vi "CODMn通讯.vi"() -> ()   [LabVIEW 2016, in "斯坦道CODMn.lvlib"]
uses:
  <vilib>/NI/Modbus Library/API/Wrapper/Create TCP Slave.vi
  <vilib>/NI/Modbus Library/API/slave/Modbus Slave.lvclass
  <vilib>/Plasmionique/MB Master/MB_Master/MB_Master.lvclass
  <vilib>/Plasmionique/MB Master/MB Master.lvlib
  <vilib>/Utility/config.llb/NI_LVConfig.lvlib
  <vilib>/NI/Modbus Library/API/Wrapper/API Main.lvlib
panel:
  out "codm程序更新":bool=TRUE
  in  "读取数据":bool
  in  "释放串口":bool
  in  "打开串口":bool
  out "队列中元素数量":i32
  out "元素":cluster{"命令":string}[](array[cluster])
  out "待处理插入数量":i32
  out "读取公式":u16[](array[numeric])
  out "读取参数":u16[](array[numeric])
  out "数据存储":u16[](array[numeric])
  out "温度":bool[](array[boolean])
  out "M输出点":bool[](array[boolean])
  out "ORP、时间":u16[](array[numeric])
  out "测量状态":u16[](array[numeric])
  out "通讯状态":bool
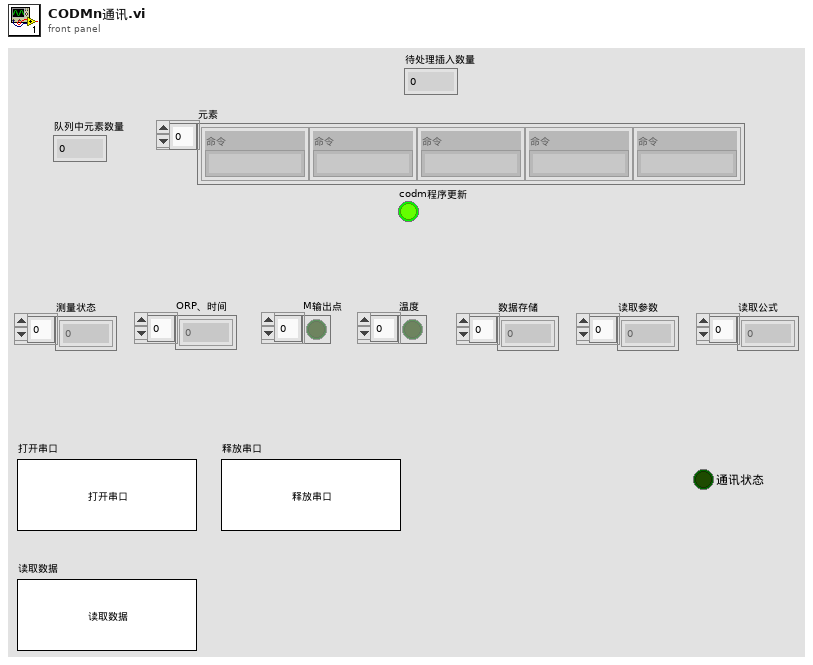
[diagram p1: front panel]
types:
  T1 = typedef "CODMn交互.ctl" = cluster{"COD浓度（mg/L)":dbl, "水样启动时间":timestamp, "加标回收启动时间":timestamp, "CODMn工作状态":enum16{"空闲", "水样测试", "标样核查", "零点核查", "跨度核查", "空白测试", "平行样测试", "加标回收", "空白校准", "标样校准", "初始化（清洗）"}, "多列列表框":i32, "平台试剂余量百分比":sgl, "关键参数":cluster{"测量量程":dbl, "测量精度":dbl, "测量间隔":dbl, "消解温度":dbl, "消解时长":dbl, "空白校准时间":timestamp, "曲线截距":dbl, "曲线斜率":dbl, "测量检出限":dbl, "测量信号值":dbl, "线性相关系数":dbl, "二次多项式系数":dbl, "标样校准时间":timestamp, "稀释倍数":dbl, "三项式系数":dbl, "空白标定系数":dbl, "量程系数":dbl, "F0/ORPA":dbl, "F1/ORPB":dbl, "F2/ORPK":dbl, "F3":dbl, "F4":dbl, "F5":dbl, "F6":dbl, "F7":dbl, "X0/滴定数":dbl, "量程":dbl}, "关键参数改变":bool, "校准信息":cluster{"低标液1浓度":dbl, "低标液1信号值":dbl, "低标液1启用":u16, "低标液2浓度":dbl, "低标液2信号值":dbl, "低标液2启用":u16, "低标液3浓度":dbl, "低标液3信号值":dbl, "低标液3启用":u16, "低标液4浓度":dbl, "低标液4信号值":dbl, "低标液4启用":u16, "低标液5浓度":dbl, "低标液5信号值":dbl, "低标液5启用":u16, "高标液1浓度":dbl, "高标液1信号值":dbl, "高标液1启用":u16, "高标液2浓度":dbl, "高标液2信号值":dbl, "高标液2启用":u16, "高标液3浓度":dbl, "高标液3信号值":dbl, "高标液3启用":u16, "高标液4浓度":dbl, "高标液4信号值":dbl, "高标液4启用":u16, "高标液5浓度":dbl, "高标液5信号值":dbl, "高标液5启用":u16}, "校准信息改变":bool}
  T2 = cluster{"测量模式":enum16{"水样测量", "标样核查", "零点核查", "跨度核查", "空白测试", "加标回收", "平行样", "校零", "校标"}}
  T3 = cluster{"命令":string, "测量模式":enum16{"水样测量", "标样核查", "零点核查", "跨度核查", "空白测试", "加标回收", "平行样", "校零", "校标"}, "CODMn量程切换":enum32{"H", "L", "AUTO"}}
  T4 = typedef "NI_LVConfig.lvlib/Config Data RefNum.ctl" = refnum<k1>
  T5 = enum16{"空闲", "水样测试", "标样核查", "零点核查", "跨度核查", "空白测试", "平行样测试", "质控样", "空白校准", "标样校准", "加标回收"}
  T6 = cluster{"测量量程":dbl, "测量精度":dbl, "测量间隔":dbl, "消解温度":dbl, "消解时长":dbl, "空白校准时间":timestamp, "曲线截距":dbl, "曲线斜率":dbl, "测量检出限":dbl, "测量信号值":dbl, "线性相关系数":dbl, "二次多项式系数":dbl, "标样校准时间":timestamp, "稀释倍数":dbl, "三项式系数":dbl, "空白标定系数":dbl, "量程系数":dbl, "F0/ORPA":dbl, "F1/ORPB":dbl, "F2/ORPK":dbl, "F3":dbl, "F4":dbl, "F5":dbl, "F6":dbl, "F7":dbl, "X0/滴定数":dbl, "量程":dbl}
  T7 = cluster{"低标液1浓度":dbl, "低标液1信号值":dbl, "低标液1启用":u16, "低标液2浓度":dbl, "低标液2信号值":dbl, "低标液2启用":u16, "低标液3浓度":dbl, "低标液3信号值":dbl, "低标液3启用":u16, "低标液4浓度":dbl, "低标液4信号值":dbl, "低标液4启用":u16, "低标液5浓度":dbl, "低标液5信号值":dbl, "低标液5启用":u16, "高标液1浓度":dbl, "高标液1信号值":dbl, "高标液1启用":u16, "高标液2浓度":dbl, "高标液2信号值":dbl, "高标液2启用":u16, "高标液3浓度":dbl, "高标液3信号值":dbl, "高标液3启用":u16, "高标液4浓度":dbl, "高标液4信号值":dbl, "高标液4启用":u16, "高标液5浓度":dbl, "高标液5信号值":dbl, "高标液5启用":u16}
  T8 = enum16{"水样测量", "标样核查", "零点核查", "跨度核查", "空白测试", "加标回收", "平行样", "校零", "校标"}
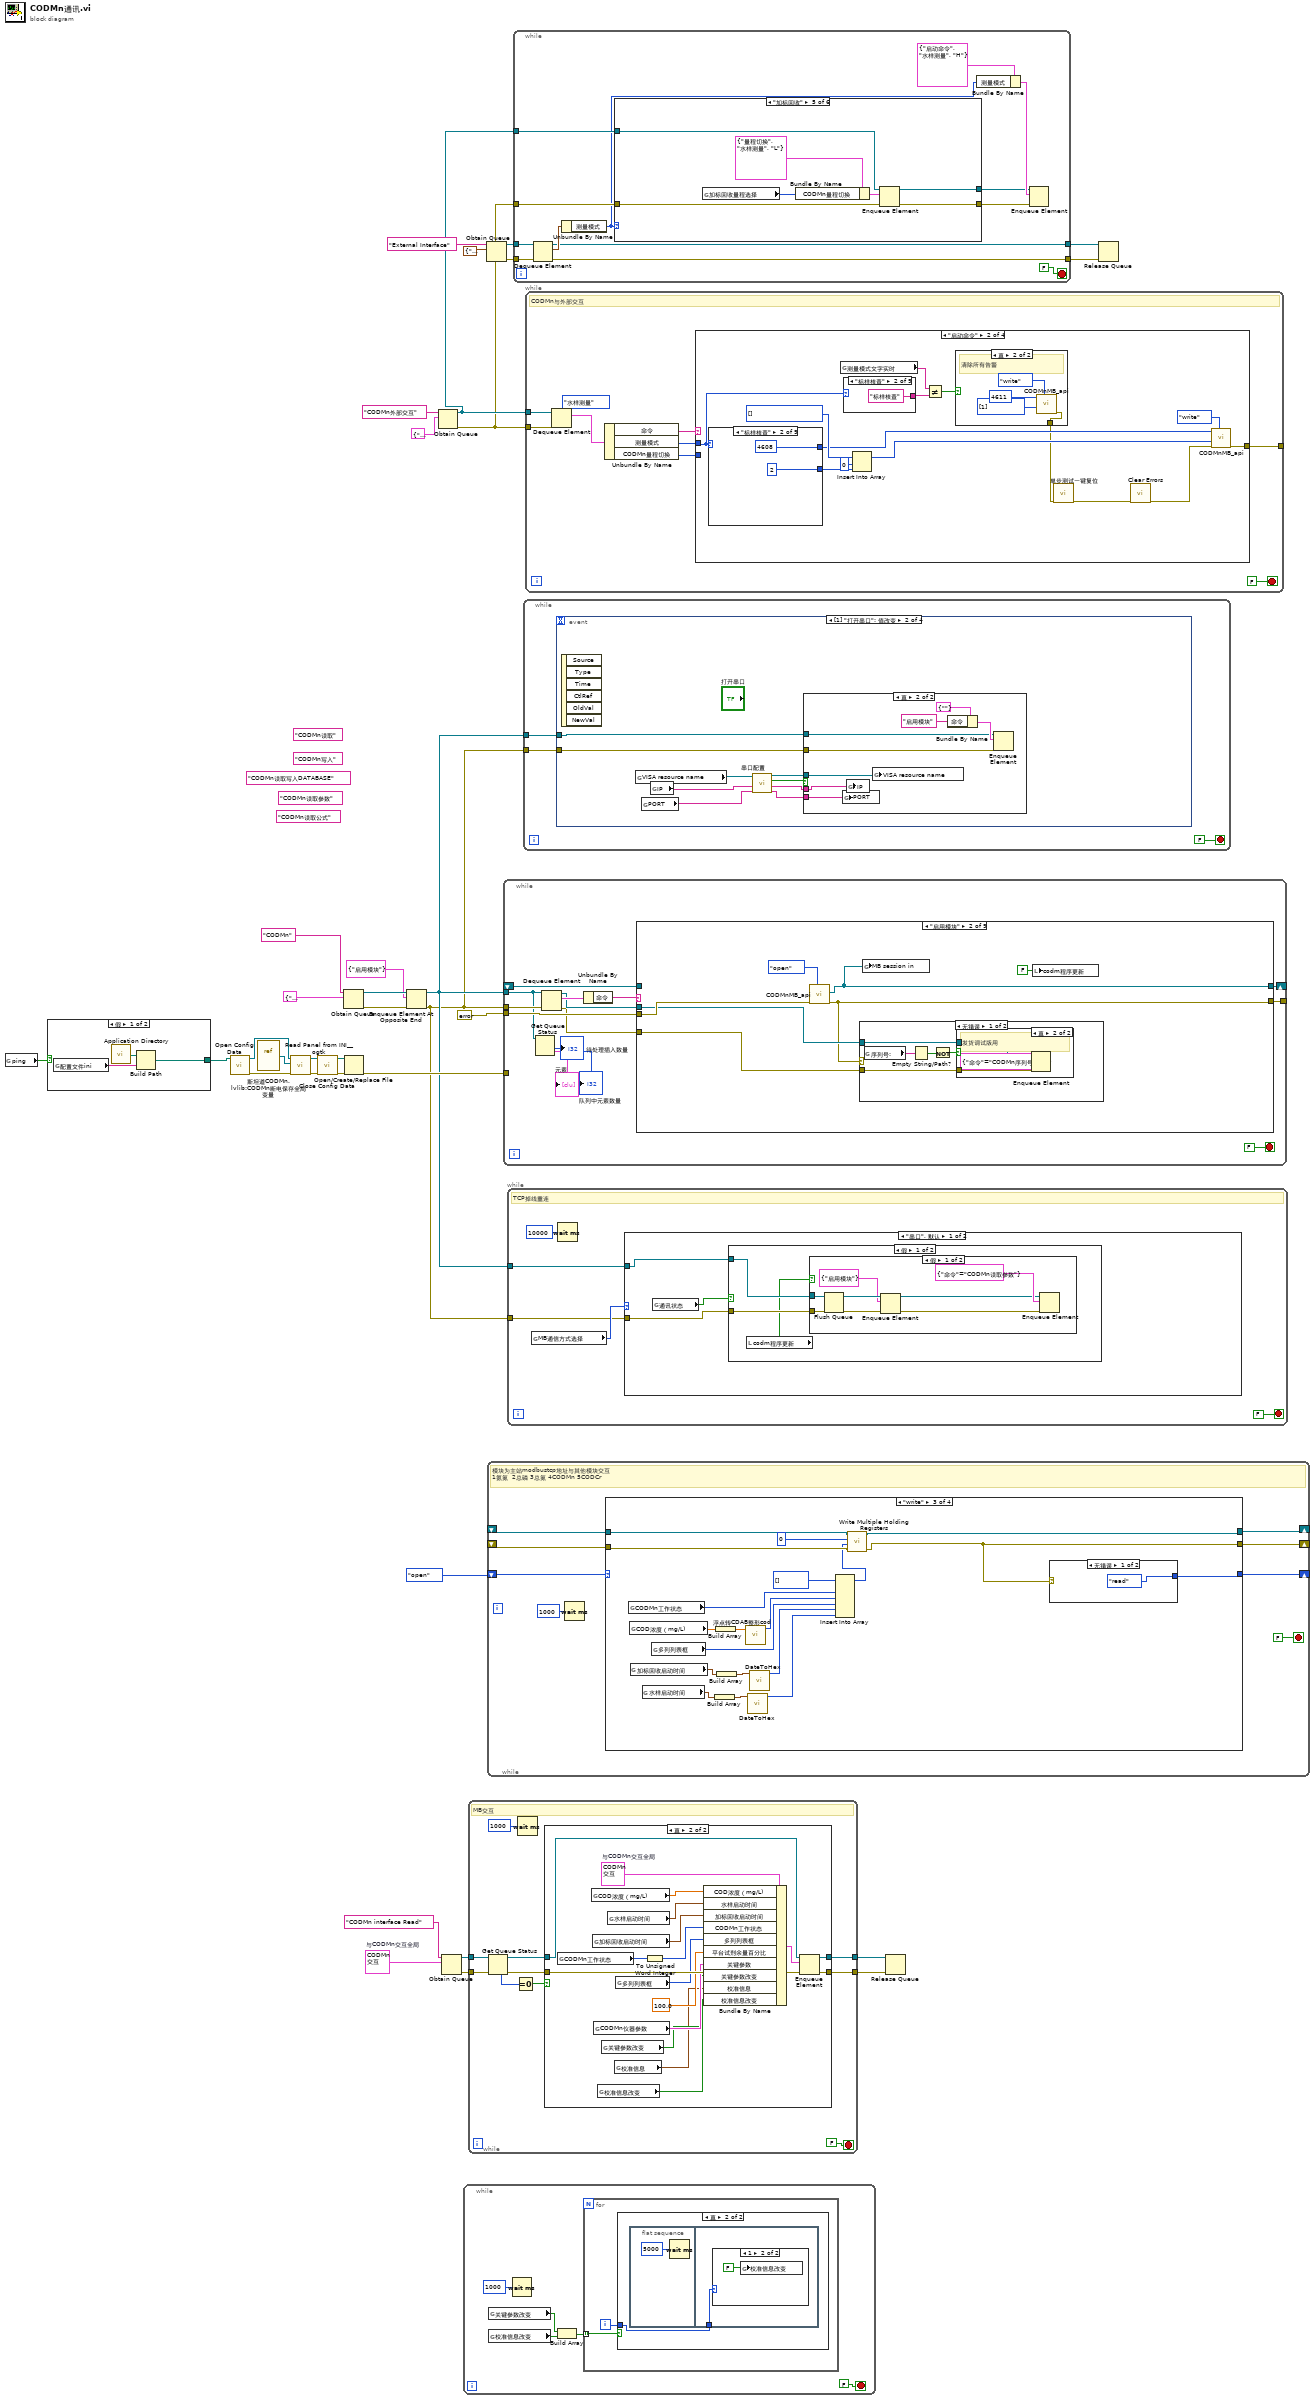
[diagram p0: block diagram]
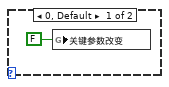
[diagram p3: hidden frame]
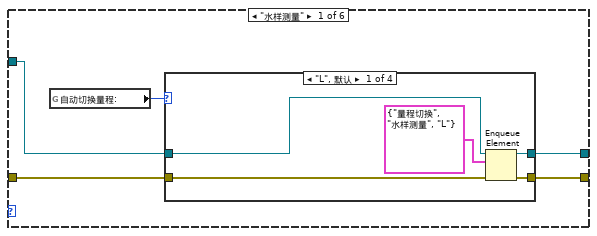
[diagram p5: hidden frame]
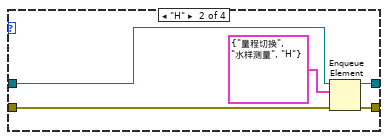
[diagram p6: hidden frame]
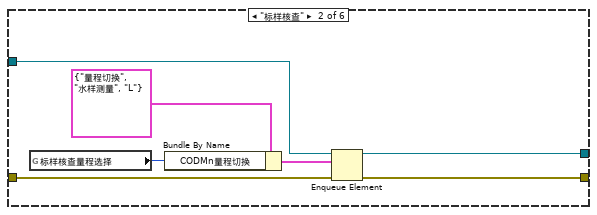
[diagram p9: hidden frame]
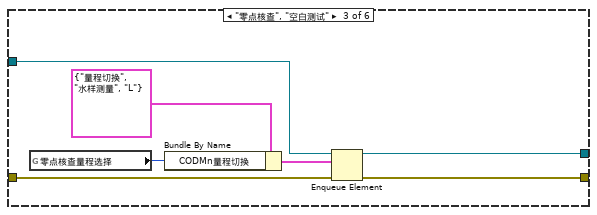
[diagram p10: hidden frame]
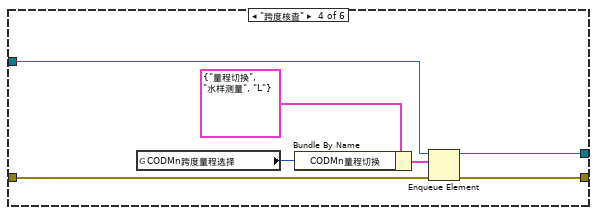
[diagram p11: hidden frame]
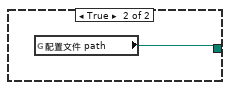
[diagram p13: hidden frame]
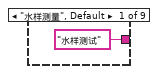
[diagram p16: hidden frame]
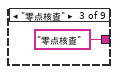
[diagram p17: hidden frame]
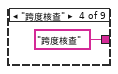
[diagram p18: hidden frame]
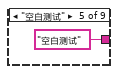
[diagram p19: hidden frame]
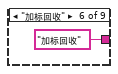
[diagram p20: hidden frame]
diagram:
  w2 = T1 {"COD浓度（mg/L)"=0.0, "水样启动时间"=timestamp(0 s since 1904-01-01), "加标回收启动时间"=timestamp(0 s since 1904-01-01), "CODMn工作状态"=enum."空闲", "多列列表框"=0, "平台试剂余量百分比"=0.0, "关键参数"={"测量量程"=0.0, "测量精度"=0.0, "测量间隔"=0.0, "消解温度"=0.0, "消解时长"=0.0, "空白校准时间"=timestamp(0 s since 1904-01-01), "曲线截距"=0.0, "曲线斜率"=0.0, "测量检出限"=0.0, "测量信号值"=0.0, "线性相关系数"=0.0, "二次多项式系数"=0.0, "标样校准时间"=timestamp(0 s since 1904-01-01), "稀释倍数"=0.0, "三项式系数"=0.0, "空白标定系数"=0.0, "量程系数"=0.0, "F0/ORPA"=0.0, "F1/ORPB"=0.0, "F2/ORPK"=0.0, "F3"=0.0, "F4"=0.0, "F5"=0.0, "F6"=0.0, "F7"=0.0, "X0/滴定数"=0.0, "量程"=0.0}, "关键参数改变"=FALSE, "校准信息"={"低标液1浓度"=0.0, "低标液1信号值"=0.0, "低标液1启用"=0, "低标液2浓度"=0.0, "低标液2信号值"=0.0, "低标液2启用"=0, "低标液3浓度"=0.0, "低标液3信号值"=0.0, "低标液3启用"=0, "低标液4浓度"=0.0, "低标液4信号值"=0.0, "低标液4启用"=0, "低标液5浓度"=0.0, "低标液5信号值"=0.0, "低标液5启用"=0, "高标液1浓度"=0.0, "高标液1信号值"=0.0, "高标液1启用"=0, "高标液2浓度"=0.0, "高标液2信号值"=0.0, "高标液2启用"=0, "高标液3浓度"=0.0, "高标液3信号值"=0.0, "高标液3启用"=0, "高标液4浓度"=0.0, "高标液4信号值"=0.0, "高标液4启用"=0, "高标液5浓度"=0.0, "高标液5信号值"=0.0, "高标液5启用"=0}, "校准信息改变"=FALSE}  # 与CODMn交互全局
  (unwired) "CODMn读取公式" ("名称（未命名）")
  (unwired) "CODMn读取写入DATABASE" ("名称（未命名）")
  (unwired) "CODMn读取参数" ("名称（未命名）")
  (unwired) "CODMn读取" ("名称（未命名）")
  (unwired) "CODMn写入" ("名称（未命名）")
  n1 = global read "CODMN外部API.vi" "ping"() -> (w17:bool)
  n2 = case shown="假" w17 {
    tunnel: [w36 w39] -> w16
    frame False {
      n3 = global read "COD内部交互全局.vi" "配置文件ini"() -> (w38:string)
      n4 = call <vilib>:"Application Directory.vi"() -> ("Application Directory"=w37:path)
      n5 = Build Path(base path=w37, name or relative path=w38) -> (appended path=w36:path)
    }
    frame True {
      n6 = global read "CODMN外部API.vi" "配置文件 path"() -> (w39:path)
    }
  }
  n7 = call <vilib>:"Open Config Data.vi"("configuration file path"=w16) -> ("error out"=w27:errorcluster, "refnum"=w30:T4)  [unwired: 8 in, 1 out]
  n8 = vi-ref "斯坦道CODMn.lvlib:CODMn断电保存全局变量.vi"() -> (w29:refnum<vi>)
  n9 = call <userlib>:"Read Panel from INI__ogtk.vi"("error in (no error)"=w27, "VI ref"=w29, "refnum"=w30) -> ("error out"=w26:errorcluster, "refnum out"=w28:T4)  [unwired: 7 in]
  n10 = call <vilib>:"Close Config Data.vi"("error in (no error)"=w26, "refnum"=w28) -> ("error out"=w25:errorcluster, "file path"=w24:path)  [unwired: 8 in]
  n11 = Obtain Queue(name (unnamed)="CODMn", element data type=cluster{"命令":string} {"命令"="启用模块"} ("元素")) -> (queue out=w33:refnum<queue>, error out=w32:errorcluster)  [unwired: 3 in, 1 out]
  n12 = Open/Create/Replace File(file path (use dialog)=w24, error in=w25) -> (error out=w23:errorcluster)  [unwired: 4 in, 2 out]
  n13 = Enqueue Element At Opposite End(queue=w33, element=cluster{"命令":string} {"命令"="启用模块"} ("元素"), error in (no error)=w32) -> (queue out=w21:refnum<queue>, error out=w20:errorcluster)  [unwired: 1 in, 1 out]
  n14 = Obtain Queue(name (unnamed)="CODMn外部交互" ("名称（未命名）"), element data type=T3 {"命令"="启动命令", "测量模式"=enum."水样测量", "CODMn量程切换"=enum."AUTO"} ("元素")) -> (queue out=w11:refnum<queue>, error out=w10:errorcluster)  [unwired: 3 in, 1 out]
  n15 = Obtain Queue(name (unnamed)="CODMn interface Read" ("写入方名称"), element data type=w2) -> (queue out=w6:refnum<queue>, error out=w5:errorcluster)  [unwired: 3 in, 1 out]
  n16 = while {
    stop <- FALSE stop-if-true
    n17 = global read "CODMn断电保存全局变量.vi" "关键参数改变"() -> (w43:bool)
    n18 = global read "CODMn断电保存全局变量.vi" "校准信息改变"() -> (w42:bool)
    n19 = Wait (ms)(milliseconds to wait=u32 1000 ("等待时间（毫秒）")) -> ()  [unwired: 1 out]
    n20 = Build Array(w43, w42) -> (w41:bool[])
    n21 = for {
      tunnel: w41 -> [w46] mode=indexing
      i -> [w45]
      n22 = case shown="真" w46 {
        tunnel: w45 -> [_ w47]
        frame False {
        }
        frame True {
          n23 = flat-sequence {
            tunnel: w47 -> [w49]
            frame #0 {
              n24 = Wait (ms)(milliseconds to wait=u32 5000 ("等待时间（毫秒）")) -> ()  [unwired: 1 out]
            }
            frame #1 {
              n25 = case shown="1" w49 {
                frame 0, Default {
                  n26 = global write "CODMn断电保存全局变量.vi" "关键参数改变"(FALSE ("关键参数改变")) -> ()
                }
                frame 1 {
                  n27 = global write "CODMn断电保存全局变量.vi" "校准信息改变"(FALSE ("关键参数改变")) -> ()
                }
              }
            }
          }
        }
      }
    }
  }
  n28 = while {
    tunnel: w6 -> [w60]
    tunnel: w5 -> [w53]
    tunnel: [w59] -> w4
    tunnel: [w58] -> w3
    stop <- FALSE stop-if-true
    # "MB交互"
    n29 = Get Queue Status(queue=w60, error in (no error)=w53) -> (queue out=w56:refnum<queue>, error out=w52:errorcluster, # elements in queue=w55:i32)  [unwired: 1 in, 5 out]
    n30 = Equal To 0?(x=w55) -> (x = 0?=w54:bool)
    n31 = Wait (ms)(milliseconds to wait=u32 1000 ("等待时间（毫秒）")) -> ()  [unwired: 1 out]
    n32 = case shown="真" w54 {
      tunnel: w56 -> [w63 w80]
      tunnel: w52 -> [w62 w79]
      tunnel: [w63 w78] -> w59
      tunnel: [w62 w77] -> w58
      frame False {
      }
      frame True {
        w76 = T1 {"COD浓度（mg/L)"=0.0, "水样启动时间"=timestamp(0 s since 1904-01-01), "加标回收启动时间"=timestamp(0 s since 1904-01-01), "CODMn工作状态"=enum."空闲", "多列列表框"=0, "平台试剂余量百分比"=0.0, "关键参数"={"测量量程"=0.0, "测量精度"=0.0, "测量间隔"=0.0, "消解温度"=0.0, "消解时长"=0.0, "空白校准时间"=timestamp(0 s since 1904-01-01), "曲线截距"=0.0, "曲线斜率"=0.0, "测量检出限"=0.0, "测量信号值"=0.0, "线性相关系数"=0.0, "二次多项式系数"=0.0, "标样校准时间"=timestamp(0 s since 1904-01-01), "稀释倍数"=0.0, "三项式系数"=0.0, "空白标定系数"=0.0, "量程系数"=0.0, "F0/ORPA"=0.0, "F1/ORPB"=0.0, "F2/ORPK"=0.0, "F3"=0.0, "F4"=0.0, "F5"=0.0, "F6"=0.0, "F7"=0.0, "X0/滴定数"=0.0, "量程"=0.0}, "关键参数改变"=FALSE, "校准信息"={"低标液1浓度"=0.0, "低标液1信号值"=0.0, "低标液1启用"=0, "低标液2浓度"=0.0, "低标液2信号值"=0.0, "低标液2启用"=0, "低标液3浓度"=0.0, "低标液3信号值"=0.0, "低标液3启用"=0, "低标液4浓度"=0.0, "低标液4信号值"=0.0, "低标液4启用"=0, "低标液5浓度"=0.0, "低标液5信号值"=0.0, "低标液5启用"=0, "高标液1浓度"=0.0, "高标液1信号值"=0.0, "高标液1启用"=0, "高标液2浓度"=0.0, "高标液2信号值"=0.0, "高标液2启用"=0, "高标液3浓度"=0.0, "高标液3信号值"=0.0, "高标液3启用"=0, "高标液4浓度"=0.0, "高标液4信号值"=0.0, "高标液4启用"=0, "高标液5浓度"=0.0, "高标液5信号值"=0.0, "高标液5启用"=0}, "校准信息改变"=FALSE}  # 与CODMn交互全局
        n33 = global read "COD测量模式全局.vi" "CODMn工作状态"() -> (w73:T5)
        n34 = global read "COD浓度全局变量.vi" "COD浓度（mg/L)"() -> (w68:dbl)
        n35 = global read "COD测量模式全局.vi" "加标回收启动时间"() -> (w72:timestamp)
        n36 = global read "CODMn断电保存全局变量.vi" "CODMn仪器参数"() -> (w75:T6)
        n37 = global read "CODMn断电保存全局变量.vi" "校准信息改变"() -> (w65:bool)
        n38 = global read "CODMn断电保存全局变量.vi" "关键参数改变"() -> (w66:bool)
        n39 = global read "COD测量模式全局.vi" "水样启动时间"() -> (w71:timestamp)
        n40 = global read "CODMn断电保存全局变量.vi" "校准信息"() -> (w64:T7)
        n41 = global read "运行时序全局变量.vi" "多列列表框"() -> (w69:i32)
        n42 = To Unsigned Word Integer(number=w73) -> (unsigned 16bit integer=w74:u16)
        n43 = Bundle By Name(cluster=w76, "COD浓度（mg/L)"=w68, "水样启动时间"=w71, "加标回收启动时间"=w72, "CODMn工作状态"=w74, "多列列表框"=w69, "平台试剂余量百分比"=sgl 100.0, "关键参数"=w75, "关键参数改变"=w66, "校准信息"=w64, "校准信息改变"=w65) -> (w67:T1)
        n44 = Enqueue Element(queue=w80, element=w67, error in (no error)=w79) -> (queue out=w78:refnum<queue>, error out=w77:errorcluster)  [unwired: 1 in, 1 out]
      }
    }
  }
  n45 = Obtain Queue(name (unnamed)="External Interface" ("名称（未命名）"), element data type=T2 {"测量模式"=enum."水样测量"} ("启动测量模式")) -> (queue out=w13:refnum<queue>, error out=w12:errorcluster)  [unwired: 3 in, 1 out]
  n46 = while {
    shift-right: [w86] -> _
    shift-left: _ -> [w88]
    shift-right: [w85] -> _
    shift-left: _ -> [w87]
    shift-right: [w82] -> _
    shift-left: enum16{"open", "read", "write", "close"}."open" -> [w83]
    stop <- FALSE stop-if-true
    # "模块为主站modbustcp地址与其他模块交互\n1氨氮  2总磷 3总氮 4CODMn 5CODCr"
    n47 = Wait (ms)(milliseconds to wait=u32 1000 ("等待时间（毫秒）")) -> ()  [unwired: 1 out]
    n48 = case shown="\"write\"" w83 {
      selector: w83 -> [w97 _ _ _]
      tunnel: w88 -> [w91 w105 w128 w134]
      tunnel: w87 -> [w90 w104 w125 w133]
      tunnel: [w94 w101 w127 w134] -> w86
      tunnel: [w93 w100 w126 w136] -> w85
      tunnel: [w96 w108 w129 enum16{"open", "read", "write", "close"}."open"] -> w82
      frame "open", Default {
        n49 = call-dynamic "Shutdown.vi"("error in"=w90, "Modbus slave in"=w91) -> ("error out"=w89:errorcluster)  [unwired: 9 in]
        n50 = call <vilib>:"Clear Errors.vi"("error in (no error)"=w89) -> ("error out"=w92:errorcluster)  [unwired: 5 in, 1 out]
        n51 = call-poly <vilib>:"Create Modbus Instance.vi"("error in"=w92, "port (502)"=u16 4) -> ("error out"=w93:errorcluster, "TCP slave instance"=w94:refnum<class "Modbus Slave.lvclass">)  [unwired: 8 in]
        n52 = case shown="错误" w93 {
          tunnel: w97 -> [_ w99]
          tunnel: [enum16{"open", "read", "write", "close"}."write" w99] -> w96
          frame No Error {
          }
          frame Error {
          }
        }
      }
      frame "read" {
        n53 = call-dynamic <vilib>:"Read Holding Registers.vi"("error in"=w104, "number of inputs"=u16 1, "starting address"=u16 257, "Modbus slave in"=w105) -> ("error out"=w100:errorcluster, "register values"=w103:u16[], "Modbus slave out"=w101:refnum<class "Modbus Slave.lvclass">)  [unwired: 5 in]
        n54 = Index Array(array=w103) -> (element=w102:u16)  [unwired: 1 in]
        n55 = global write "CODMN外部API.vi" "CODMn状态"(w102) -> ()
        n56 = case shown="无错误" w100 {
          tunnel: [enum16{"open", "read", "write", "close"}."write" enum16{"open", "read", "write", "close"}."close"] -> w108
          frame No Error {
          }
          frame Error {
          }
        }
      }
      frame "write" {
        n57 = global read "COD测量模式全局.vi" "CODMn工作状态"() -> (w115:T5)
        n58 = global read "COD浓度全局变量.vi" "COD浓度（mg/L)"() -> (w117:dbl)
        n59 = global read "COD测量模式全局.vi" "加标回收启动时间"() -> (w120:timestamp)
        n60 = global read "COD测量模式全局.vi" "水样启动时间"() -> (w122:timestamp)
        n61 = global read "运行时序全局变量.vi" "多列列表框"() -> (w119:i32)
        n62 = Build Array(w122) -> (w121:timestamp[])
        n63 = Build Array(w117) -> (w116:dbl[])
        n64 = Build Array(w120) -> (w113:timestamp[])
        n65 = call "浮点转CDAB整形cod.vi"("浮点数"=w116) -> ("CDAB整形输出"=w118:u16[])  [unwired: 10 in]
        n66 = call "DateToHex.vi"("DATE"=w121) -> ("数组"=w124:u16[])  [unwired: 10 in]
        n67 = call "DateToHex.vi"("DATE"=w113) -> ("数组"=w123:u16[])  [unwired: 10 in]
        n68 = Insert Into Array(array=u16[] [] ("values"), new element #1=w115, new element #2=w118, new element #3=w119, new element #4=w123, new element #5=w124) -> (w112:u16[])  [unwired: 1 in]
        n69 = call-dynamic "Write Multiple Holding Registers.vi"("error in"=w125, "registers to write"=w112, "starting address"=u16 0, "Modbus slave in"=w128) -> ("error out"=w126:errorcluster, "Modbus slave out"=w127:refnum<class "Modbus Slave.lvclass">)  [unwired: 6 in]
        n70 = case shown="无错误" w126 {
          tunnel: [enum16{"open", "read", "write", "close"}."read" enum16{"open", "read", "write", "close"}."close"] -> w129
          frame No Error {
          }
          frame Error {
          }
        }
      }
      frame "close" {
        n71 = call-dynamic "Shutdown.vi"("error in"=w133, "Modbus slave in"=w134) -> ("error out"=w132:errorcluster)  [unwired: 9 in]
        n72 = call <vilib>:"Clear Errors.vi"("error in (no error)"=w132) -> ("error out"=w136:errorcluster)  [unwired: 5 in, 1 out]
      }
    }
  }
  n73 = while {
    tunnel: w21 -> [w142]
    tunnel: w20 -> [w149]
    tunnel: [w143] -> _
    shift-right: [w146] -> _
    shift-left: _ -> [w145]
    tunnel: errorcluster {"status"=FALSE, "code"=0, "source"=""} ("error out") -> [w144]
    tunnel: w23 -> [_]
    stop <- FALSE stop-if-true
    n74 = Get Queue Status(queue=w142) -> (# pending insert=→"待处理插入数量":i32, # elements in queue=→"队列中元素数量":i32, elements=→"元素":cluster{"命令":string}[])  [unwired: 2 in, 5 out]
    n75 = Dequeue Element(queue=w142, error in (no error)=w149) -> (queue out=w138:refnum<queue>, element=w148:cluster{"命令":string}, error out=w137:errorcluster)  [unwired: 1 in, 1 out]
    n76 = Unbundle By Name(w148) -> ("命令"=w147:string)
    n77 = case shown="\"启用模块\"" w147 {
      tunnel: [w152 w157 w169 w177 w209 w218 w235 w242 w249] -> w146
      tunnel: [w151 w154 w170 w174 w207 w217 w234 w241 w248] -> w143
      tunnel: w145 -> [w152 _ _ w201 w213 w227 w238 w246 w252]
      tunnel: w144 -> [w151 w158 w171 w200 w210 w226 w237 w245 w250]
      tunnel: w138 -> [_ w156 _ _ _ _ _ _ _]
      tunnel: w137 -> [_ w155 _ _ _ _ _ _ _]
      frame Default {
      }
      frame "启用模块" {
        n78 = call "CODMnMB_api.vi"("STEP"=enum16{"open", "read", "write", "close"}."open", "Error in"=w158) -> ("error out"=w154:errorcluster, "MB session out"=w157:refnum<class "MB_Master.lvclass">)  [unwired: 7 in, 1 out]
        n79 = case shown="无错误" w154 {
          tunnel: w156 -> [w164 _]
          tunnel: w155 -> [w163 _]
          frame No Error {
            n80 = global read "COD内部交互全局.vi" "序列号:"() -> (w162:string)
            n81 = Empty String/Path?(string/path=w162) -> (empty?=w161:bool)
            n82 = Not(x=w161) -> (.not. x?=w160:bool)
            n83 = case shown="真" w160 {
              tunnel: w164 -> [_ w167]
              tunnel: w163 -> [_ w166]
              frame False {
              }
              frame True {
                # "发货调试版用"
                n84 = Enqueue Element(queue=w167, element=cluster{"命令":string} {"命令"="CODMn序列号写入"} ("元素"), error in (no error)=w166) -> ()  [unwired: 1 in, 3 out]
              }
            }
          }
          frame Error {
          }
        }
        n85 = global write "COD浓度全局变量.vi" "MB session in"(w157) -> ()
        n86 = local write "codm程序更新"(FALSE ("codm程序更新")) -> ()
      }
      frame "停用模块" {
        n87 = call "CODMnMB_api.vi"("STEP"=enum16{"open", "read", "write", "close"}."close", "Error in"=w171) -> ("error out"=w170:errorcluster, "MB session out"=w169:refnum<class "MB_Master.lvclass">)  [unwired: 7 in, 1 out]
        "codm程序更新" <- TRUE
      }
      frame "CODMn读取" {
        n88 = call <vilib>:"Read Holding Registers.vi"("error in (no error)"=w200, "quantity"=u16 50 ("number of holding registers"), "starting address"=u16 4224, "MB session in"=w201) -> ("error out"=w191:errorcluster, "Registers"=w197:u16[], "MB session out"=w192:refnum<class "MB_Master.lvclass">)  [unwired: 5 in]
        n89 = case shown="无错误" w191 {
          tunnel: w197 -> [w206 _]
          frame No Error {
            n90 = global write "COD内部交互全局.vi" "测量状态"(w206) -> ()
            "测量状态" <- w206
          }
          frame Error {
          }
        }
        n91 = call <vilib>:"Read Holding Registers.vi"("error in (no error)"=w191, "quantity"=u16 10, "starting address"=u16 4101, "MB session in"=w192) -> ("error out"=w187:errorcluster, "Registers"=w190:u16[], "MB session out"=w189:refnum<class "MB_Master.lvclass">)  [unwired: 5 in]
        n92 = case shown="无错误" w187 {
          tunnel: w190 -> [w205 _]
          frame No Error {
            n93 = global write "COD内部交互全局.vi" "ORP、时间"(w205) -> ()
            "ORP、时间" <- w205
          }
          frame Error {
          }
        }
        n94 = call <vilib>:"Read Coils.vi"("error in (no error)"=w187, "quantity"=u16 11, "starting address"=u16 137, "MB session in"=w189) -> ("error out"=w185:errorcluster, "Coils"=w186:bool[], "MB session out"=w188:refnum<class "MB_Master.lvclass">)  [unwired: 5 in]
        n95 = case shown="无错误" w185 {
          tunnel: w186 -> [w204 _]
          frame No Error {
            n96 = global write "COD内部交互全局.vi" "M输出点"(w204) -> ()
            "M输出点" <- w204
          }
          frame Error {
          }
        }
        n97 = call <vilib>:"Read Coils.vi"("error in (no error)"=w185, "quantity"=u16 1, "starting address"=u16 400, "MB session in"=w188) -> ("error out"=w178:errorcluster, "Coils"=w182:bool[], "MB session out"=w179:refnum<class "MB_Master.lvclass">)  [unwired: 5 in]
        n98 = case shown="无错误" w178 {
          tunnel: w182 -> [w203 _]
          frame No Error {
            n99 = global write "COD内部交互全局.vi" "温度"(w203) -> ()
            "温度" <- w203
          }
          frame Error {
          }
        }
        n100 = call <vilib>:"Read Coils.vi"("error in (no error)"=w178, "quantity"=u16 20, "starting address"=u16 500, "MB session in"=w179) -> ("error out"=w174:errorcluster, "Coils"=w173:bool[], "MB session out"=w177:refnum<class "MB_Master.lvclass">)  [unwired: 5 in]
        n101 = case shown="无错误" w174 {
          tunnel: w173 -> [w202 _]
          frame No Error {
            n102 = global write "COD内部交互全局.vi" "报警点位"(w202) -> ()
          }
          frame Error {
          }
        }
        n103 = Unbundle By Name(w174) -> ("status"=w181:bool)
        n104 = Not(x=w181) -> (.not. x?=w180:bool)
        "通讯状态" <- w180
        n105 = global write "COD内部交互全局.vi" "通讯状态"(w180) -> ()
      }
      frame "CODMn读取写入DATABASE" {
        n106 = call <vilib>:"Read Holding Registers.vi"("error in (no error)"=w210, "quantity"=u16 10 ("number of holding registers"), "starting address"=u16 4101, "MB session in"=w213) -> ("error out"=w207:errorcluster, "Registers"=w208:u16[], "MB session out"=w209:refnum<class "MB_Master.lvclass">)  [unwired: 5 in]
        n107 = case shown="无错误" w207 {
          tunnel: w208 -> [w215 _]
          frame No Error {
            n108 = global write "COD内部交互全局.vi" "数据存储"(w215) -> ()
            n109 = global write "COD内部交互全局.vi" "读取写入data"(TRUE ("读取参数显示")) -> ()
            "数据存储" <- w215
          }
          frame Error {
          }
        }
      }
      frame "CODMn读取参数" {
        n110 = call <vilib>:"Read Holding Registers.vi"("error in (no error)"=w226, "quantity"=u16 35 ("number of holding registers"), "starting address"=u16 4272, "MB session in"=w227) -> ("error out"=w221:errorcluster, "Registers"=w223:u16[], "MB session out"=w222:refnum<class "MB_Master.lvclass">)  [unwired: 5 in]
        n111 = case shown="无错误" w221 {
          tunnel: w223 -> [w231 _]
          frame No Error {
            n112 = global write "COD内部交互全局.vi" "读取参数"(w231) -> ()
            n113 = global write "COD内部交互全局.vi" "读取参数显示"(TRUE ("读取参数显示")) -> ()
            "读取参数" <- w231
          }
          frame Error {
          }
        }
        n114 = call <vilib>:"Read Holding Registers.vi"("error in (no error)"=w221, "quantity"=u16 4, "starting address"=u16 5596, "MB session in"=w222) -> ("error out"=w217:errorcluster, "Registers"=w216:u16[], "MB session out"=w218:refnum<class "MB_Master.lvclass">)  [unwired: 5 in]
        n115 = case shown="无错误" w217 {
          tunnel: w216 -> [w229 _]
          frame No Error {
            n116 = global write "COD内部交互全局.vi" "读取浮台参数"(w229) -> ()
            n117 = global write "COD内部交互全局.vi" "读取浮台参数显示"(TRUE ("读取参数显示")) -> ()
          }
          frame Error {
          }
        }
      }
      frame "CODMn读取公式" {
        n118 = call <vilib>:"Read Holding Registers.vi"("error in (no error)"=w237, "quantity"=u16 94 ("number of holding registers"), "starting address"=u16 4616, "MB session in"=w238) -> ("error out"=w234:errorcluster, "Registers"=w236:u16[], "MB session out"=w235:refnum<class "MB_Master.lvclass">)  [unwired: 5 in]
        n119 = case shown="无错误" w234 {
          tunnel: w236 -> [w240 _]
          frame No Error {
            n120 = global write "COD内部交互全局.vi" "读取公式"(w240) -> ()
            n121 = global write "COD内部交互全局.vi" "读取公式显示"(TRUE ("读取参数显示")) -> ()
            "读取公式" <- w240
          }
          frame Error {
          }
        }
      }
      frame "CODMn序列号写入" {
        n122 = global read "COD内部交互全局.vi" "序列号:"() -> (w244:string)
        n123 = call "StringToHex.vi"("STRING"=w244) -> ("数组"=w243:u16[])  [unwired: 10 in]
        n124 = call <vilib>:"Write Multiple Registers.vi"("error in (no error)"=w245, "values"=w243, "starting address"=u16 4298, "MB session in"=w246) -> ("error out"=w241:errorcluster, "MB session out"=w242:refnum<class "MB_Master.lvclass">)  [unwired: 6 in]
      }
      frame "CODMn程序更新" {
        n125 = call <vilib>:"Write Multiple Registers.vi"("error in (no error)"=w250, "values"=u16[] [0], "starting address"=u16 4296, "MB session in"=w252) -> ("error out"=w248:errorcluster, "MB session out"=w249:refnum<class "MB_Master.lvclass">)  [unwired: 6 in]
      }
    }
  }
  n126 = while "While循环" {
    tunnel: w21 -> [w255]
    tunnel: w20 -> [w254]
    stop <- FALSE stop-if-true
    # "TCP掉线重连"
    n127 = global read "CODMn断电保存全局变量.vi" "MB通信方式选择"() -> (w256:enum16{"串口", "TCP"})
    n128 = Wait (ms)(milliseconds to wait=u32 10000 ("等待时间（毫秒）")) -> ()  [unwired: 1 out]
    n129 = case shown="\"串口\", 默认" w256 {
      tunnel: w255 -> [w260 w274]
      tunnel: w254 -> [w259 w273]
      frame "串口", Default {
        n130 = global read "COD内部交互全局.vi" "通讯状态"() -> (w261:bool)
        n131 = case shown="假" w261 {
          tunnel: w260 -> [w264 _]
          tunnel: w259 -> [w263 _]
          frame False {
            n132 = local read "codm程序更新"() -> (w262:bool)
            n133 = case shown="假" w262 {
              tunnel: w264 -> [w269 _]
              tunnel: w263 -> [w268 _]
              frame False {
                n134 = Flush Queue(queue=w269, error in (no error)=w268) -> (queue out=w272:refnum<queue>, error out=w271:errorcluster)  [unwired: 1 out]
                n135 = Enqueue Element(queue=w272, element=cluster{"命令":string} {"命令"="启用模块"} ("元素"), error in (no error)=w271) -> (queue out=w266:refnum<queue>, error out=w265:errorcluster)  [unwired: 1 in, 1 out]
                n136 = Enqueue Element(queue=w266, element=cluster{"命令":string} {"命令"="CODMn读取参数"} ("元素"), error in (no error)=w265) -> ()  [unwired: 1 in, 3 out]
              }
              frame True {
              }
            }
          }
          frame True {
          }
        }
      }
      frame "TCP" {
        n137 = global read "COD浓度全局变量.vi" "MB session in"() -> (w276:refnum<class "MB_Master.lvclass">)
        n138 = property class="MB_Master"(reference=w276) -> ("Properties:Session Valid"=w275:bool)  [unwired: 1 in, 2 out]
        n139 = case shown="假" w275 {
          tunnel: w274 -> [w281 _]
          tunnel: w273 -> [w280 _]
          frame False {
            n140 = Flush Queue(queue=w281, error in (no error)=w280) -> (queue out=w284:refnum<queue>, error out=w283:errorcluster)  [unwired: 1 out]
            n141 = Enqueue Element(queue=w284, element=cluster{"命令":string} {"命令"="启用模块"} ("元素"), error in (no error)=w283) -> (queue out=w278:refnum<queue>, error out=w277:errorcluster)  [unwired: 1 in, 1 out]
            n142 = Enqueue Element(queue=w278, element=cluster{"命令":string} {"命令"="CODMn读取参数"} ("元素"), error in (no error)=w277) -> ()  [unwired: 1 in, 3 out]
          }
          frame True {
          }
        }
      }
    }
  }
  n143 = while {
    tunnel: w13 -> [w297]
    tunnel: w12 -> [w296]
    tunnel: w11 -> [w293]
    tunnel: w10 -> [w292]
    tunnel: [w286] -> w9
    tunnel: [w285] -> w8
    stop <- FALSE stop-if-true
    n144 = Dequeue Element(queue=w297, error in (no error)=w296) -> (queue out=w286:refnum<queue>, element=w294:T2, error out=w285:errorcluster)  [unwired: 1 in, 1 out]
    n145 = Unbundle By Name(w294) -> ("测量模式"=w289:T8)
    n146 = case "条件结构" shown="\"加标回收\"" w289 {
      tunnel: w293 -> [w301 w320 w327 w334 w341 w346]
      tunnel: w292 -> [w299 w319 w326 w333 w340 w345]
      tunnel: [w300 w318 w325 w332 w339 w346] -> w288
      tunnel: [w298 w317 w324 w331 w338 w345] -> w287
      frame "水样测量" {
        n147 = global read "CODMn断电保存全局变量.vi" "自动切换量程:"() -> (w302:enum16{"L", "H", "自动切换测一次", "自动切换测两次"})
        n148 = case shown="\"L\", 默认" w302 {
          tunnel: w301 -> [w306 w312 w313 w316]
          tunnel: [w304 w311 w313 w316] -> w300
          tunnel: w299 -> [w305 w310 w314 w315]
          tunnel: [w303 w309 w314 w315] -> w298
          frame "L", Default {
            n149 = Enqueue Element(queue=w306, element=T3 {"命令"="量程切换", "测量模式"=enum."水样测量", "CODMn量程切换"=enum."L"} ("元素"), error in (no error)=w305) -> (queue out=w304:refnum<queue>, error out=w303:errorcluster)  [unwired: 1 in, 1 out]
          }
          frame "H" {
            n150 = Enqueue Element(queue=w312, element=T3 {"命令"="量程切换", "测量模式"=enum."水样测量", "CODMn量程切换"=enum."H"} ("元素"), error in (no error)=w310) -> (queue out=w311:refnum<queue>, error out=w309:errorcluster)  [unwired: 1 in, 1 out]
          }
          frame "自动切换测一次" {
          }
          frame "自动切换测两次" {
          }
        }
      }
      frame "标样核查" {
        n151 = global read "CODMn断电保存全局变量.vi" "标样核查量程选择"() -> (w322:enum32{"H", "L", "AUTO"})
        n152 = Bundle By Name(cluster=T3 {"命令"="量程切换", "测量模式"=enum."水样测量", "CODMn量程切换"=enum."L"} ("元素"), "CODMn量程切换"=w322) -> (w323:T3)
        n153 = Enqueue Element(queue=w320, element=w323, error in (no error)=w319) -> (queue out=w318:refnum<queue>, error out=w317:errorcluster)  [unwired: 1 in, 1 out]
      }
      frame "零点核查", "空白测试" {
        n154 = global read "CODMn断电保存全局变量.vi" "零点核查量程选择"() -> (w329:enum32{"H", "L", "AUTO"})
        n155 = Bundle By Name(cluster=T3 {"命令"="量程切换", "测量模式"=enum."水样测量", "CODMn量程切换"=enum."L"} ("元素"), "CODMn量程切换"=w329) -> (w328:T3)
        n156 = Enqueue Element(queue=w327, element=w328, error in (no error)=w326) -> (queue out=w325:refnum<queue>, error out=w324:errorcluster)  [unwired: 1 in, 1 out]
      }
      frame "跨度核查" {
        n157 = global read "CODMn断电保存全局变量.vi" "CODMn跨度量程选择"() -> (w336:enum32{"H", "L", "AUTO"})
        n158 = Bundle By Name(cluster=T3 {"命令"="量程切换", "测量模式"=enum."水样测量", "CODMn量程切换"=enum."L"} ("元素"), "CODMn量程切换"=w336) -> (w335:T3)
        n159 = Enqueue Element(queue=w334, element=w335, error in (no error)=w333) -> (queue out=w332:refnum<queue>, error out=w331:errorcluster)  [unwired: 1 in, 1 out]
      }
      frame "加标回收" {
        n160 = global read "CODMn断电保存全局变量.vi" "加标回收量程选择"() -> (w343:enum32{"H", "L", "AUTO"})
        n161 = Bundle By Name(cluster=T3 {"命令"="量程切换", "测量模式"=enum."水样测量", "CODMn量程切换"=enum."L"} ("元素"), "CODMn量程切换"=w343) -> (w342:T3)
        n162 = Enqueue Element(queue=w341, element=w342, error in (no error)=w340) -> (queue out=w339:refnum<queue>, error out=w338:errorcluster)  [unwired: 1 in, 1 out]
      }
      frame Default {
        # "不切换量程"
      }
    }
    n163 = Bundle By Name(cluster=T3 {"命令"="启动命令", "测量模式"=enum."水样测量", "CODMn量程切换"=enum."H"} ("元素"), "测量模式"=w289) -> (w290:T3)
    n164 = Enqueue Element(queue=w288, element=w290, error in (no error)=w287) -> ()  [unwired: 1 in, 3 out]
  }
  n165 = while {
    tunnel: w21 -> [w348]
    tunnel: w20 -> [w347]
    stop <- FALSE stop-if-true
    n166 = event shown="[1] \"打开串口\": 值改变" {
      selector: _ -> [_ _ _ _]
      dyn-events: _ -> [_ _ _ _]
      timeout: _ -> [_ _ _ _]
      tunnel: w348 -> [_ w355 w369 w371]
      tunnel: w347 -> [_ w354 w368 w370]
      event Timeout {
        n167 = event-data() -> ()  [unwired: 1 in, 3 out]
      }
      event "打开串口": Value Change {
        n168 = event-data() -> ()  [unwired: 1 in, 6 out]
        n169 = global read "CODMn断电保存全局变量.vi" "VISA resource name"() -> (w358:refnum<visa-resource-name>)
        n170 = global read "CODMn断电保存全局变量.vi" "PORT"() -> (w350:string)
        n171 = global read "CODMn断电保存全局变量.vi" "IP"() -> (w351:string)
        n172 = call "串口配置.vi"("PORT"=w350, "IP"=w351, "请选择串口:"=w358) -> ("PORT 2"=w352:string, "IP 2"=w353:string, "确认 2"=w356:bool, "VISA资源名称 2"=w357:refnum<visa-resource-name>)  [unwired: 4 in, 1 out]
        n173 = case shown="真" w356 {
          tunnel: w357 -> [_ w366]
          tunnel: w355 -> [_ w362]
          tunnel: w354 -> [_ w361]
          tunnel: w353 -> [_ w360]
          tunnel: w352 -> [_ w359]
          frame False {
          }
          frame True {
            n174 = global write "CODMn断电保存全局变量.vi" "PORT"(w359) -> ()
            n175 = global write "CODMn断电保存全局变量.vi" "IP"(w360) -> ()
            n176 = global write "CODMn断电保存全局变量.vi" "VISA resource name"(w366) -> ()
            n177 = Bundle By Name(cluster=cluster{"命令":string} {"命令"=""} ("元素"), "命令"="启用模块" ("名称（未命名）")) -> (w363:cluster{"命令":string})
            n178 = Enqueue Element(queue=w362, element=w363, error in (no error)=w361) -> ()  [unwired: 1 in, 3 out]
          }
        }
      }
      event "释放串口": Value Change {
        n179 = event-data() -> ()  [unwired: 1 in, 6 out]
        n180 = Enqueue Element(queue=w369, element=cluster{"命令":string} {"命令"="停用模块"} ("元素"), error in (no error)=w368) -> ()  [unwired: 1 in, 3 out]
      }
      event "读取数据": Value Change {
        n181 = event-data() -> ()  [unwired: 1 in, 6 out]
        n182 = Enqueue Element(queue=w371, element=cluster{"命令":string} {"命令"="CODMn读取"} ("元素"), error in (no error)=w370) -> ()  [unwired: 1 in, 3 out]
      }
    }
  }
  n183 = while {
    tunnel: w11 -> [w378]
    tunnel: w10 -> [w377]
    tunnel: [w373] -> _
    stop <- FALSE stop-if-true
    (unwired) T8."水样测量" ("测量模式")
    # "CODMn与外部交互"
    n184 = Dequeue Element(queue=w378, error in (no error)=w377) -> (element=w379:T3)  [unwired: 1 in, 3 out]
    n185 = Unbundle By Name(w379) -> ("命令"=w376:string, "测量模式"=w375:T8, "CODMn量程切换"=w374:enum32{"H", "L", "AUTO"})
    n186 = case shown="\"启动命令\"" w376 {
      tunnel: w375 -> [_ w383 _ _]
      tunnel: w374 -> [_ _ _ w433]
      tunnel: [_ w388 w428 w432] -> w373
      frame "假", Default {
      }
      frame "启动命令" {
        n187 = case shown="\"标样核查\"" w383 {
          tunnel: [u16 4608 ("address") u16 4608 ("address") u16 4608 ("address") u16 4608 ("address") u16 4608 ("address") u16 4608 ("address") u16 4608 ("address") u16 4608 ("address") u16 4608 ("address")] -> w390
          tunnel: [u16 1 ("address") u16 2 ("address") u16 3 ("address") u16 4 ("address") u16 5 ("address") u16 7 ("address") u16 6 ("address") u16 8 ("address") u16 9 ("address")] -> w394
          frame "水样测量" {
          }
          frame "标样核查" {
          }
          frame "零点核查" {
          }
          frame "跨度核查" {
          }
          frame "空白测试" {
          }
          frame "加标回收" {
          }
          frame "平行样" {
          }
          frame "校零" {
            n188 = global write "CODMN外部API.vi" "远程反控校零CODMn"(TRUE ("远程反控校准CODMn")) -> ()
          }
          frame "校标" {
            n189 = global write "CODMN外部API.vi" "远程反控校准CODMn"(TRUE ("远程反控校准CODMn")) -> ()
          }
        }
        n190 = global read "COD测量模式全局.vi" "测量模式文字实时"() -> (w384:string)
        n191 = case shown="\"标样核查\"" w383 {
          tunnel: ["水样测试" ("测量模式") "标样核查" ("测量模式") "零点核查" ("测量模式") "跨度核查" ("测量模式") "空白测试" ("测量模式") "加标回收" ("测量模式") "平行样" ("测量模式") "校零" ("测量模式") "校标" ("测量模式")] -> w385
          frame "水样测量", Default {
          }
          frame "标样核查" {
          }
          frame "零点核查" {
          }
          frame "跨度核查" {
          }
          frame "空白测试" {
          }
          frame "加标回收" {
          }
          frame "平行样" {
          }
          frame "校零" {
          }
          frame "校标" {
          }
        }
        n192 = Insert Into Array(array=u16[] [] ("values"), index=0 ("索引"), new element=w394) -> (w389:u16[])
        n193 = Not Equal?(x=w384, y=w385) -> (x != y?=w382:bool)
        n194 = case shown="真" w382 {
          tunnel: [_ w395] -> w381
          frame False {
          }
          frame True {
            # "清除所有告警"
            n195 = call "CODMnMB_api.vi"("STEP"=enum16{"open", "read", "write", "close"}."write", "values"=u16[] [1], "starting address"=u16 4611) -> ("error out"=w395:errorcluster)  [unwired: 6 in, 2 out]
          }
        }
        n196 = call "单步测试一键复位.vi"("Error in"=w381) -> ("error out"=w387:errorcluster)  [unwired: 10 in]
        n197 = call <vilib>:"Clear Errors.vi"("error in (no error)"=w387) -> ("error out"=w386:errorcluster)  [unwired: 5 in, 1 out]
        n198 = call "CODMnMB_api.vi"("STEP"=enum16{"open", "read", "write", "close"}."write", "Error in"=w386, "values"=w389, "starting address"=w390) -> ("error out"=w388:errorcluster)  [unwired: 5 in, 2 out]
      }
      frame "停止命令" {
        n199 = call "CODMnMB_api.vi"("STEP"=enum16{"open", "read", "write", "close"}."write", "values"=u16[] [11], "starting address"=u16 4608) -> ("error out"=w428:errorcluster)  [unwired: 6 in, 2 out]
      }
      frame "量程切换" {
        n200 = case shown="\"H\"" w433 {
          tunnel: [u16[] [1] ("values") u16[] [0] ("values") _] -> w436
          frame "H" {
          }
          frame "L" {
          }
          frame "AUTO", Default {
          }
        }
        n201 = call "CODMnMB_api.vi"("STEP"=enum16{"open", "read", "write", "close"}."write", "values"=w436, "starting address"=u16 4276) -> ("error out"=w432:errorcluster)  [unwired: 6 in, 2 out]
      }
    }
  }
  n202 = Release Queue(queue=w4, error in (no error)=w3) -> ()  [unwired: 1 in, 3 out]
  n203 = Release Queue(queue=w9, error in (no error)=w8) -> ()  [unwired: 1 in, 3 out]
